vi "4_DMA_1Msps.vi"() -> ()   [LabVIEW 2015]
uses:
  <vilib>/Instr/_visa.llb/VISA Configure Serial Port (Instr).vi
panel:
  in  "VISA resource name":refnum<visa-resource-name>="COM7"
  out "error out":errorcluster={"status"=TRUE, "code"=-1073807343, "source"="VISA Open in 4_DMA_1Msps.vi"}
  out "Measurement":u8[](graph)
  in  "stop":bool
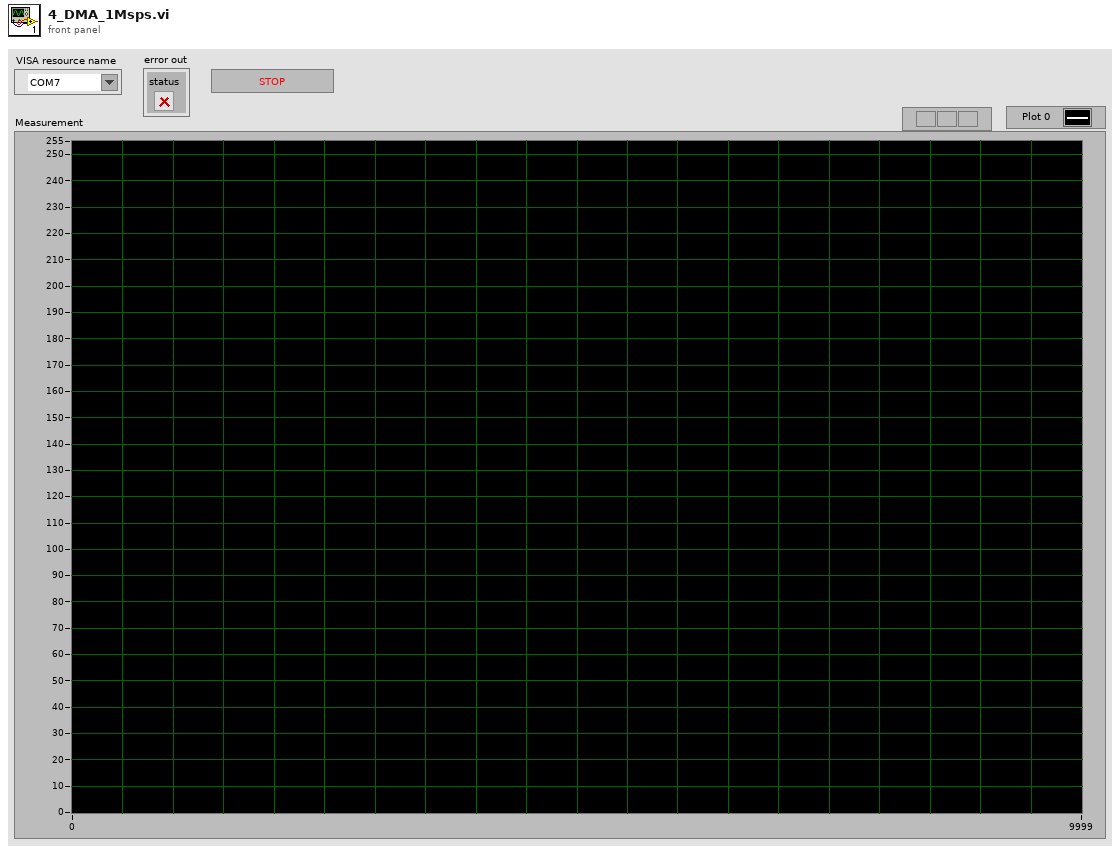
[diagram p1: front panel]
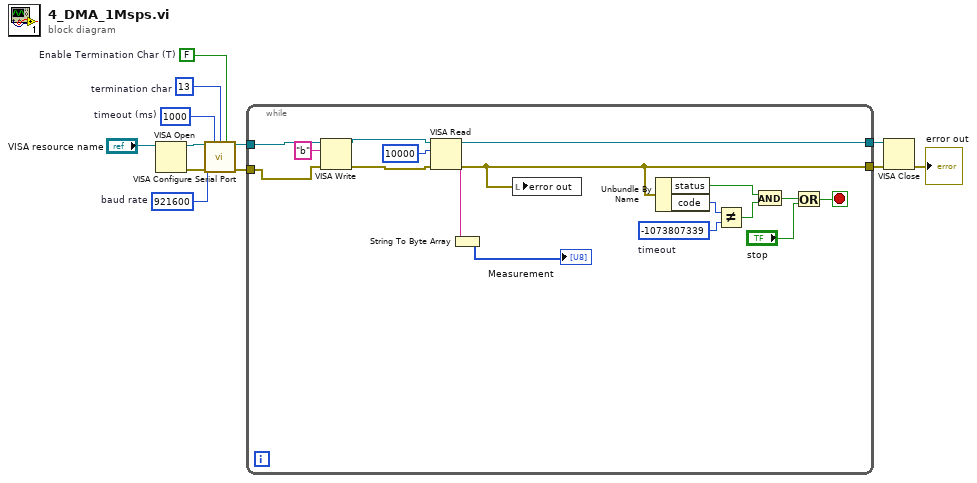
[diagram p0: block diagram]
diagram:
  w1 = u32 921600  # baud rate
  w2 = u32 1000  # timeout (ms)
  w8 = FALSE  # Enable Termination Char (T)
  w9 = u8 13  # termination char
  n1 = VISA Open(VISA resource name="VISA resource name") -> (VISA resource name=w11:refnum<visa-resource-name>, error out=w12:errorcluster)  [unwired: 4 in]
  n2 = call-poly "VISA Configure Serial Port"("VISA resource name"=w11, "timeout (10sec)"=w2, "termination char\n(0xA = '\\n' = LF)"=w9, "Enable Termination\nChar (T)"=w8, "baud rate (9600)"=w1, "error in (no error)"=w12) -> ("VISA resource name out"=w5:refnum<visa-resource-name>, "error out"=w4:errorcluster)  [unwired: 8 in]
  n3 = while {
    tunnel: w5 -> [w28]
    tunnel: [w29] -> w7
    tunnel: w4 -> [w27]
    tunnel: [w23] -> w6
    stop <- w17 stop-if-true
    w21 = -1073807339  # timeout
    n4 = VISA Write(VISA resource name=w28, write buffer="b", error in (no error)=w27) -> (VISA resource name out=w25:refnum<visa-resource-name>, error out=w24:errorcluster)  [unwired: 1 out]
    n5 = VISA Read(VISA resource name=w25, byte count=u32 10000, error in (no error)=w24) -> (VISA resource name out=w29:refnum<visa-resource-name>, read buffer=w15:string, error out=w23:errorcluster)  [unwired: 1 out]
    n6 = String To Byte Array(string=w15) -> (unsigned byte array=→"Measurement":u8[])
    n7 = local write "error out"(w23) -> ()
    n8 = Unbundle By Name(w23) -> ("status"=w19:bool, "code"=w22:i32)
    n9 = Not Equal?(x=w22, y=w21) -> (x != y?=w20:bool)
    n10 = And(x=w19, y=w20) -> (x .and. y?=w18:bool)
    n11 = Or(x=w18, y="stop") -> (x .or. y?=w17:bool)
  }
  n12 = VISA Close(VISA resource name=w7, error in (no error)=w6) -> (error out=→"error out":errorcluster)
